vi "DMA Output StatusMod.vi"(8 "error in (no error)":errorcluster, 11 "Refnum in":refnum<k20>) -> (0 "error out":errorcluster, 1 "dma fullness":u32, 2 "underflows":u32, 3 "Refnum out":refnum<k20>, 5 "empty elements":u32)   [LabVIEW 2017]
uses:
  <vilib>/Utility/error.llb/Error Cluster From Error Code.vi
  <vilib>/rvi/errors/niLvFpgaAdjustHostInterfaceError.vi
  <vilib>/rvi/interface/nirviMethod/nirviMethod.xnode
  <vilib>/rvi/interface/nirviReadWriteControl/nirviReadWriteControl.xnode
  <vilib>/FPGAPlugInAG/Dynamic/niLvFpga_AcquireWriteRegionFifo_Dynamic.vi
  <vilib>/rvi/errors/niLvFpgaMergeErrorWithErrorCode.vi
  NiFpgaLv.dll
  <vilib>/rvi/interface/Simulation/niFpgaSimulationCallBeginRW.vi
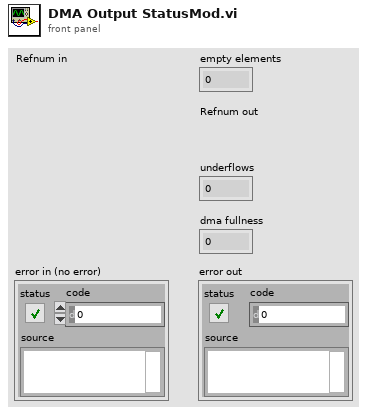
[diagram p1: front panel]
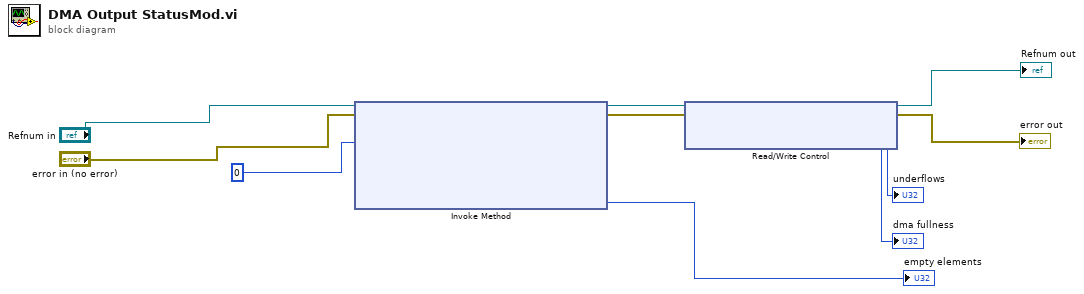
[diagram p0: block diagram]
diagram:
  n1 = xnode "Invoke Method"("FPGA VI Reference In"="Refnum in", "error in"="error in (no error)", "Number of Elements"=u32 0) -> ("FPGA VI Reference Out"=w2:refnum<k20>, "error out"=w1:errorcluster, "Empty Elements Remaining"=→"empty elements":u32)  [unwired: 1 in, 2 out]
  n2 = xnode "Read/Write Control"("FPGA VI Reference In"=w2, "error in"=w1) -> ("FPGA VI Reference Out"=→"Refnum out":refnum<k20>, "error out"=→"error out":errorcluster, "streaming output.dma min elements"=→"underflows":u32, "streaming output.dma fullness"=→"dma fullness":u32)
